vi "Set Readout Rate.vi"(8 "error in (no error)":errorcluster, 11 "CCDCamera in":refnum<class "iKon-L.lvclass">) -> (0 "error out":errorcluster, 3 "CCDCamera out":refnum<class "iKon-L.lvclass">)   [LabVIEW 2018, in "iKon-L.lvclass"]
doc: "Set readout rate"
uses:
  iKon-L.lvclass
  C:/Users/Denis/Desktop/S4ACS/S4ACS/Sim_CCD/Sim_CCD.lvclass
  Sim_CCD/Sim_CCD.lvclass
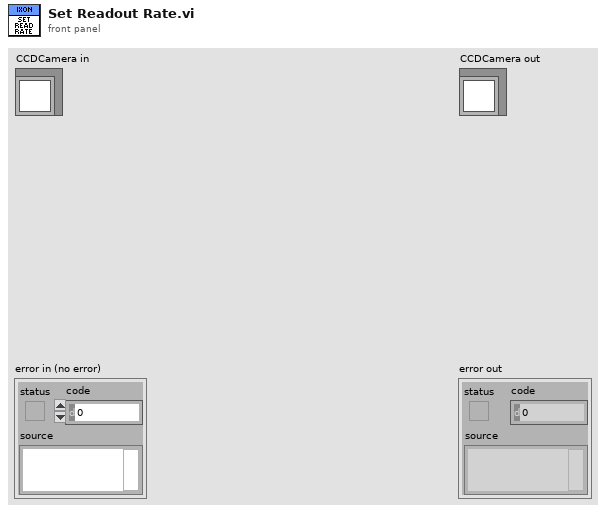
[diagram p1: front panel]
types:
  T1 = cluster{"PREAMP":u16, "READOUT_RATE":u16, "VERTICAL_SHIFT_SPEED":u16, "READ_MODE":u16, "VERTICAL_CLOCK_VOLTAGE":u16, "ACQUISITION_MODE":u16, "AD_CHANNEL":u16, "SHUTTER_TTL":u16, "SHUTTER_OPENING_TIME":u16, "SHUTTER_CLOSING_TIME":u16, "SHUTTER_MODE":u16, "TRIGGER_MODE":u16, "VBIN":u16, "INITIAL_LINE":u16, "INITIAL_COLUMN":u16, "FINAL_LINE":u16, "FINAL_COLUMN":u16, "HBIN":u16}
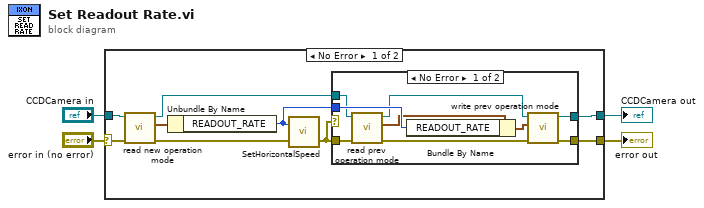
[diagram p0: block diagram]
diagram:
  n1 = case shown="No Error" "error in (no error)" {
    selector: "error in (no error)" -> [w11 w26]
    tunnel: [w13 w26] -> w4
    tunnel: [w8 w25] -> w3
    tunnel: "CCDCamera in" -> [w12 w25]
    frame No Error {
      n2 = call "read new operation mode.vi"("error in (no error)"=w11, "CCDCamera in"=w12) -> ("error out"=w6:errorcluster, "new operation mode"=w10:T1, "CCDCamera out"=w9:refnum<class "iKon-L.lvclass">)  [unwired: 7 in]
      n3 = Unbundle By Name(w10) -> ("READOUT_RATE"=w5:u16)
      n4 = call <userlib>:"SetHorizontalSpeed.vi"("error in (no error)"=w6, "index"=w5) -> ("error out"=w7:errorcluster)  [unwired: 1 out]
      n5 = case shown="No Error" w7 {
        tunnel: [w17 w24] -> w13
        tunnel: w5 -> [w22 _]
        tunnel: w7 -> [w21 w24]
        tunnel: w9 -> [w15 w23]
        tunnel: [w18 w23] -> w8
        frame No Error {
          n6 = call "read prev operation mode.vi"("error in (no error)"=w21, "Simulated_CCD_Camera in"=w15) -> ("error out"=w16:errorcluster, "prev operation mode"=w20:T1, "Simulated_CCD_Camera out"=w14:refnum<class "iKon-L.lvclass">)  [unwired: 7 in]
          n7 = Bundle By Name(cluster=w20, "READOUT_RATE"=w22) -> (w19:T1)
          n8 = call "write prev operation mode.vi"("error in (no error)"=w16, "prev operation mode"=w19, "Simulated_CCD_Camera in"=w14) -> ("error out"=w17:errorcluster, "Simulated_CCD_Camera out"=w18:refnum<class "iKon-L.lvclass">)  [unwired: 7 in]
        }
        frame Error {
        }
      }
    }
    frame Error {
    }
  }
  "error out" <- w4
  "CCDCamera out" <- w3
